vi "h5_osc_save.vi"(4 "Waveform Data":waveform(dbl)[](graph)=[{"t0"=timestamp(0 s since 1904-01-01), "dt"=6e-09, "Y"=array[1000 elements]}, {"t0"=timestamp(0 s since 1904-01-01), "dt"=6e-09, "Y"=array[1000 elements]}], 5 "Scope":cluster{"Manufacturer":string, "Model":string}={"Manufacturer"="Skynet", "Model"="T1000"}, 7 "TYPE":string="OSC_#", 8 "Bin size":i16, 9 "Settings":T1[](array[typedef])=[{"channel name"="CHANNEL1", "probe attenuation"=0.0, "vertical offset"=0.0, "vertical range"=0.0, "vertical coupling"=1, "input impedance"=0.0}, {"channel name"="CHANNEL2", "probe attenuation"=1.0, "vertical offset"=0.0, "vertical range"=1.0, "vertical coupling"=1, "input impedance"=50.0}] {"input impedance" format="%#_13g"; "vertical coupling" items=["AC", "DC", "GND"]; "vertical range" format="%.3f"; "vertical offset" format="%.3f"; "probe attenuation" format="%.3f"}, 10 "SQUID":string="100", 11 "H5":path[](array[path])=[path ""]) -> (0 "error out":errorcluster)   [LabVIEW 2015]
uses:
  osc_channel.ctl
  <vilib>/UPVI/lvhdf5/dataset.llb/LVH5D Operation.ctl
  <vilib>/UPVI/lvhdf5/dataset.llb/Simple OpenCreateReplace Dataset (Variant).vi
  <vilib>/Utility/VariantDataType/GetClusterInfo.vi
  <vilib>/Utility/VariantDataType/GetTypeInfo.vi
  <vilib>/UPVI/lvhdf5/attribute.llb/Write Multiple Attributes.vi
  <vilib>/UPVI/lvhdf5/dataset.llb/Append Element(s) to Dataset (Variant).vi
  <vilib>/UPVI/lvhdf5/dataset.llb/Simple OpenCreateReplace Dataset.xnode
  <vilib>/UPVI/lvhdf5/library.llb/HDF5 Ref.ctl
  <vilib>/UPVI/lvhdf5/attribute.llb/LVH5A Operation.ctl
  <vilib>/UPVI/lvhdf5/attribute.llb/LVH5 Write Attributes.xnode
  <vilib>/UPVI/lvhdf5/attribute.llb/Cluster to Attribute Array.xnode
  <vilib>/UPVI/lvhdf5/dataset.llb/Append Element(s) to Dataset.xnode
  oskar_tools/oskar_tools.lvlib
  <vilib>/Utility/VariantDataType/VariantType.lvlib
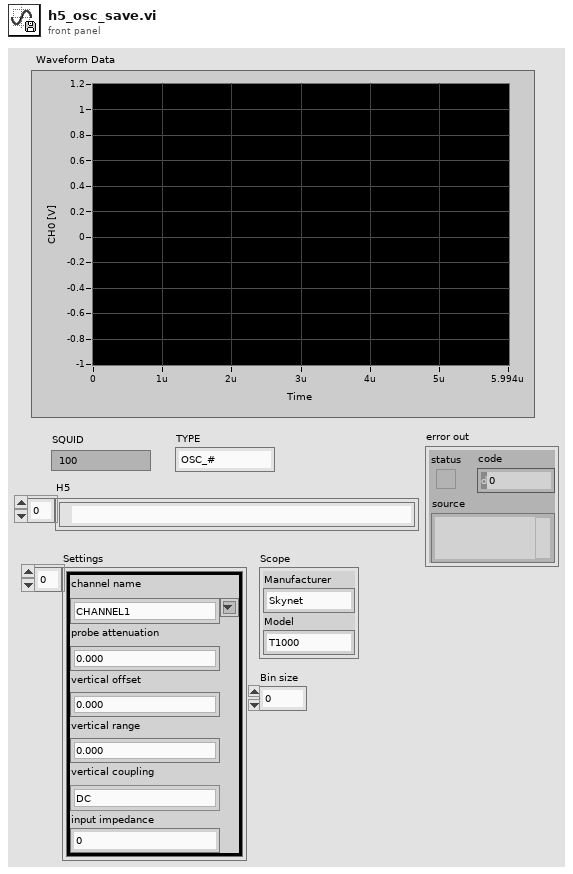
[diagram p1: front panel]
types:
  T1 = typedef "osc_channel.ctl" = cluster{"channel name":string, "probe attenuation":dbl, "vertical offset":dbl, "vertical range":dbl, "vertical coupling":i32, "input impedance":dbl}
  T2 = typedef "Semaphore RefNum" = refnum<k1>
  T3 = typedef "LVH5D Operation.ctl" = enum16{"open", "replace", "create", "open or create", "create or replace", "create or replace with confirmation"}
  T4 = typedef "HDF5 Ref.ctl" = refnum<k1>
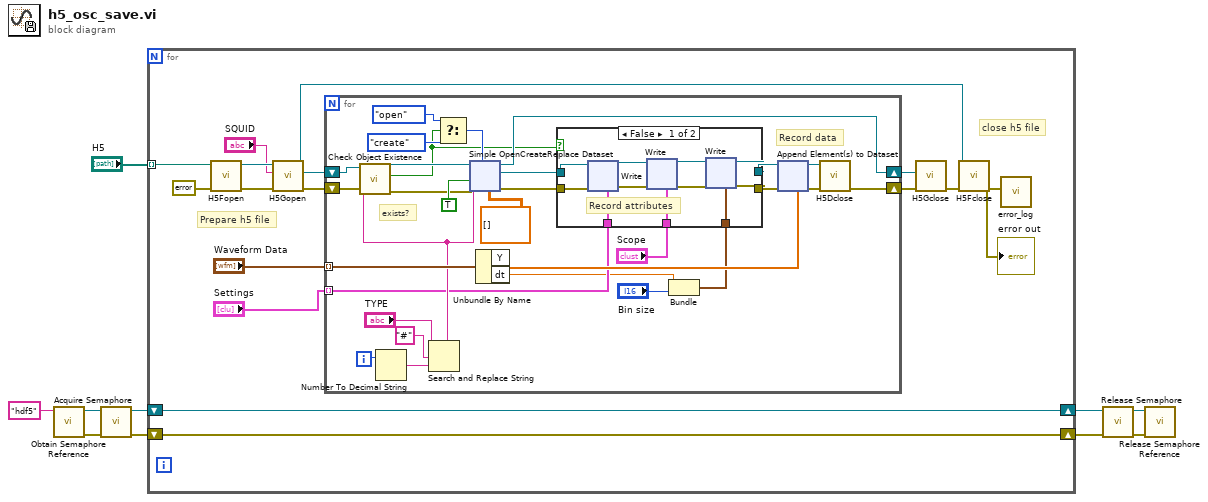
[diagram p0: block diagram]
diagram:
  n1 = call <vilib>:"Obtain Semaphore Reference.vi"("name (unnamed)"="hdf5") -> ("error out"=w8:errorcluster, "semaphore"=w9:T2)  [unwired: 4 in, 1 out]
  n2 = call <vilib>:"Acquire Semaphore.vi"("error in (no error)"=w8, "semaphore"=w9) -> ("error out"=w3:errorcluster, "semaphore out"=w4:T2)  [unwired: 3 in, 1 out]
  n3 = for {
    tunnel: "H5" -> [w24] mode=indexing
    shift-right: [w25] -> w2
    shift-left: w4 -> [w25]
    shift-right: [w26] -> w1
    shift-left: w3 -> [w26]
    # "close h5 file"
    # "Prepare h5 file"
    n4 = call <vilib>:"H5Fopen.vi"("error in (no error)"=errorcluster {"status"=FALSE, "code"=0, "source"=""} ("error out"), "path"=w24) -> ("error out"=w22:errorcluster, "HDF5 Ref out"=w21:T4)  [unwired: 6 in]
    n5 = call <vilib>:"H5Gopen.vi"("error in (no error)"=w22, "Name"="SQUID", "HDF5 Ref"=w21) -> ("error out"=w15:errorcluster, "HDF5 Group Ref"=w16:T4, "HDF5 Ref out"=w19:T4)  [unwired: 4 in]
    n6 = for {
      tunnel: "Waveform Data" -> [w55] mode=indexing
      shift-right: [w49] -> w13
      shift-left: w16 -> [w44]
      shift-right: [w50] -> w14
      shift-left: w15 -> [w42]
      tunnel: "Settings" -> [w36] mode=indexing
      i -> [w45]
      # "exists?"
      # "Record data"
      n7 = Number To Decimal String(number=w45) -> (decimal integer string=w48:string)  [unwired: 1 in]
      n8 = Search and Replace String(input string="TYPE", search string="#", replace string=w48) -> (result string=w43:string)  [unwired: 5 in, 3 out]
      n9 = call <vilib>:"Check Object Existence.vi"("error in (no error)"=w42, "name"=w43, "HDF5 Ref"=w44) -> ("error out"=w41:errorcluster, "Exists"=w32:bool, "HDF5 Ref out"=w40:T4)  [unwired: 4 in]
      n10 = Select(t=LVH5D_Operation."open" ("operation"), s=w32, f=LVH5D_Operation."create" ("operation")) -> (s? t:f=w37:T3)
      n11 = xnode "Simple OpenCreateReplace Dataset"("Dataset Path"=w43, "HDF5 Ref"=w40, "Unlimited  dataset (F)"=TRUE, "error in (no error)"=w41, "operation"=w37, "Datatype and Dataspace"=dbl[][] []) -> ("HDF5 Dataset Ref out"=w31:T4, "HDF5 Ref out"=w49:T4, "error out"=w35:errorcluster)  [unwired: 2 in]
      n12 = Unbundle By Name(w55) -> ("Y"=w54:dbl[], "dt"=w28:dbl)
      n13 = Bundle("dt"=w28, "Bin size"="Bin size") -> (w27:cluster{"dt":dbl, "Bin size":i16})  [unwired: 1 in]
      n14 = case shown="False" w32 {
        tunnel: w36 -> [w67 _]
        tunnel: w35 -> [w66 w425]
        tunnel: [w57 w425] -> w34
        tunnel: [w58 w424] -> w33
        tunnel: w31 -> [w65 w424]
        tunnel: "Scope" -> [w64 _]
        tunnel: w27 -> [w60 _]
        frame False {
          # "Record attributes"
          n15 = xnode "Write"("HDF5 Ref"=w65, "error in (no error)"=w66, "Value(s)"=w67) -> ("HDF5 Ref out"=w62:T4, "error out"=w63:errorcluster)  [unwired: 2 in]
          n16 = xnode "Write"("HDF5 Ref"=w62, "error in (no error)"=w63, "Value(s)"=w64) -> ("HDF5 Ref out"=w59:T4, "error out"=w61:errorcluster)  [unwired: 2 in]
          n17 = xnode "Write"("HDF5 Ref"=w59, "error in (no error)"=w61, "Value(s)"=w60) -> ("HDF5 Ref out"=w58:T4, "error out"=w57:errorcluster)  [unwired: 2 in]
        }
        frame True {
        }
      }
      n18 = xnode "Append Element(s) to Dataset"("HDF5 Dataset Ref"=w33, "error in (no error)"=w34, "Data Element(s)"=w54) -> ("HDF5 Dataset out"=w51:T4, "error out"=w52:errorcluster)  [unwired: 1 in, 2 out]
      n19 = call <vilib>:"H5Dclose.vi"("error in (no error)"=w52, "HDF5 Dataset Ref"=w51) -> ("error out"=w50:errorcluster)  [unwired: 7 in]
    }
    n20 = call <vilib>:"H5Gclose.vi"("error in (no error)"=w14, "HDF5 Group Ref"=w13) -> ("error out"=w20:errorcluster)  [unwired: 7 in]
    n21 = call <vilib>:"H5Fclose.vi"("error in (no error)"=w20, "HDF5 Ref"=w19) -> ("error out"=w18:errorcluster)  [unwired: 7 in]
    "error out" <- w18
    n22 = call "error_log.vi"("error"=w18) -> ()  [unwired: 10 in]
  }
  n23 = call <vilib>:"Release Semaphore.vi"("error in (no error)"=w1, "semaphore"=w2) -> ("error out"=w6:errorcluster, "semaphore out"=w5:T2)  [unwired: 4 in]
  n24 = call <vilib>:"Release Semaphore Reference.vi"("error in (no error)"=w6, "semaphore"=w5) -> ()  [unwired: 8 in, 2 out]
